vi "Draw Actor Core UI on SubPanel.vi"(8 "error in (no error)":errorcluster, 11 "Panel Manager in":refnum<class "Panel Manager.lvclass">) -> (0 "error out":errorcluster, 3 "Panel Manager out":refnum<class "Panel Manager.lvclass">)   [LabVIEW 2020, in "Panel Manager.lvclass"]
uses:
  Panel Manager.lvclass
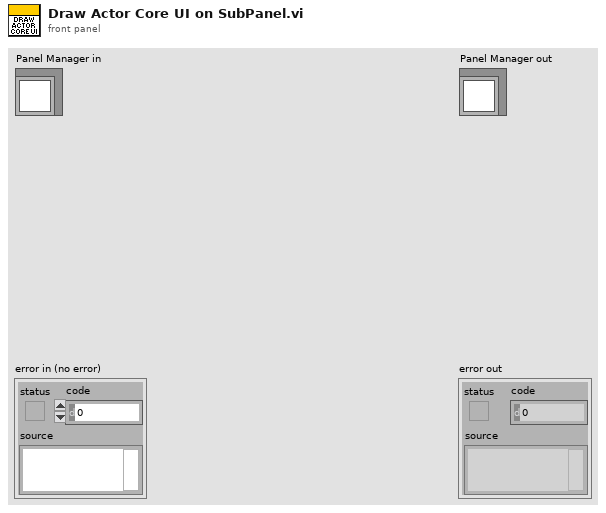
[diagram p1: front panel]
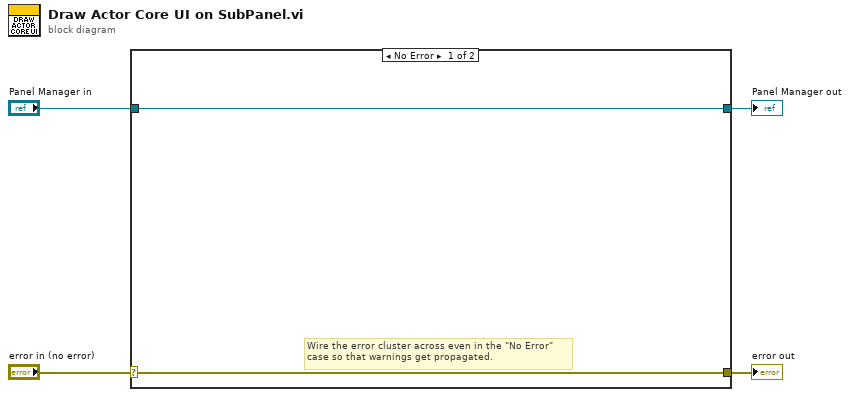
[diagram p0: block diagram]
diagram:
  n1 = case shown="No Error" "error in (no error)" {
    selector: "error in (no error)" -> [w5 w8]
    tunnel: [w5 w8] -> w3
    tunnel: [w6 w7] -> w1
    tunnel: "Panel Manager in" -> [w6 w7]
    frame No Error {
      # "Wire the error cluster across even in the \"No Error\"\ncase so that warnings get propagated."
    }
    frame Error {
    }
  }
  "error out" <- w3
  "Panel Manager out" <- w1
